vi "Test Copy Image Greyscale Mask ARGB.vi"(8 "error in (no error)":errorcluster, 11 "Test Case In":refnum<class "Image.lvclass">) -> (0 "error out":errorcluster, 3 "Test Case Out":refnum<class "Image.lvclass">)   [LabVIEW 2020, in "g_ar_toolkit.test.lvlib" / "Image.lvclass"]
uses:
  Image.lvclass
  C:/Program Files (x86)/National Instruments/LabVIEW 2020/vi.lib/Astemes/LUnit/Test Case.lvclass
  g_ar_toolkit.common/Image Size (Integer).ctl
  <vilib>/Astemes/LUnit/Test Case.lvclass/Test Case.ctl
  g_ar_toolkit.image/CreateEmptyImageGreyscale.vi
  g_ar_toolkit.image/CopyArrayToImageGreyscale.vi
  g_ar_toolkit.image/CreateEmptyImageARGB.vi
  g_ar_toolkit.image/CopyImageGreyscaleMaskARGB.vi
  4993e8ee-a06a-463a-9684-69129f64d5ce.vi
  g_ar_toolkit.image/CopyArrayToImageARGB.vi
  g_ar_toolkit.image/CreateEmptyImageGreyscale.vi/6598b9e0-8a08-46f5-91fd-ca1b87217137.vi
  g_ar_toolkit.image/CopyArrayToImageGreyscale.vi/26c70cee-9332-41f4-9755-08948a885cbe.vi
  g_ar_toolkit.image/CreateEmptyImageARGB.vi/3321fa97-f432-4e1e-8db9-a0df79aed21b.vi
  g_ar_toolkit.image/CopyImageGreyscaleMaskARGB.vi/327a14ae-2acc-4952-87c0-fab6c3cd3da3.vi
  <vilib>/Astemes/LUnit/Append Pass Result.vi
  <vilib>/Astemes/LUnit/Append Fail Result.vi
  <vilib>/Astemes/LUnit/Describe Comparison.vi
  <vilib>/Astemes/LUnit/Compare Variants.vi
  g_ar_toolkit.image/CopyArrayToImageARGB.vi/26c70cee-9332-41f4-9755-08948a885cbe.vi
  <vilib>/Astemes/LUnit/Run In UI.vi
  <vilib>/Utility/error.llb/Clear Errors.vi
  g_ar_toolkit.image/ARGBColourToU32.vi
  g_ar_toolkit.common/Module Path.vi
  <vilib>/Utility/error.llb/Error Cluster From Error Code.vi
  <vilib>/picture/pixmap.llb/Flatten Pixmap.vi
  <vilib>/Astemes/LUnit/Describe Variant.vi
  Image.lvclass/Image.ctl
  g_ar_toolkit.image/g_ar_toolkit.image.lvlib
  g_ar_toolkit.common/g_ar_toolkit.common.lvlib
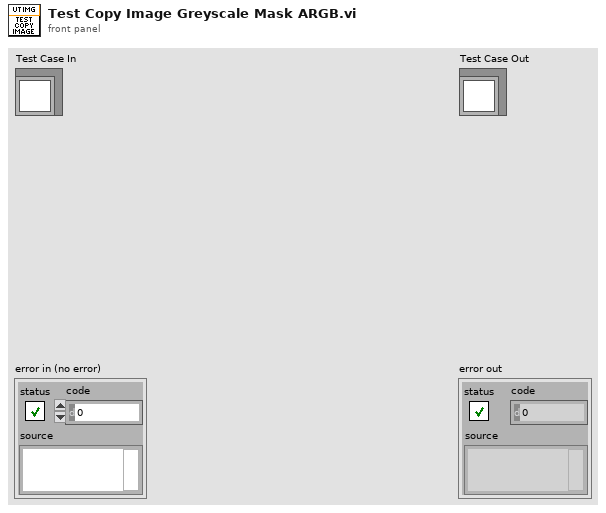
[diagram p1: front panel]
types:
  T1 = typedef "g_ar_toolkit.common.lvlib/Image Size (Integer).ctl" = cluster{"Width":u16, "Height":u16}
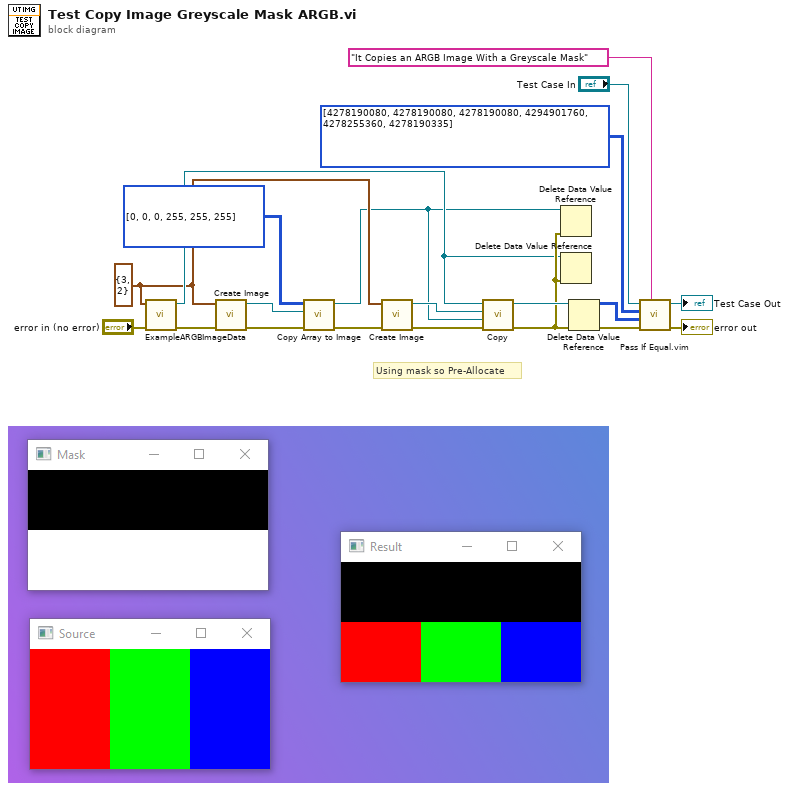
[diagram p0: block diagram]
diagram:
  w7 = T1 {"Width"=3, "Height"=2} ("Preallocated Image Size (Default - 0,0)")
  # "Using mask so Pre-Allocate"
  n1 = call "ExampleARGBImageData.vi"("error in (no error)"="error in (no error)", "Image Size"=w7) -> ("error out"=w11:errorcluster, "Data Value Reference out"=w8:refnum<data-value>)  [unwired: 6 in, 2 out]
  n2 = call-poly "Create Image.vi"("error in (no error)"=w11, "Preallocated Image Size (Default 0,0)"=w7) -> ("error out"=w15:errorcluster, "New Greyscale Image"=w4:refnum<data-value>)  [unwired: 8 in]
  n3 = call-poly "Copy Array to Image.vi"("error in (no error)"=w15, "Greyscale Destination Image"=w4, "Source"=u8[][] [[0, 0, 0], [255, 255, 255]]) -> ("error out"=w6:errorcluster, "Greyscale Destination Image (duplicate)"=w3:refnum<data-value>)  [unwired: 7 in]
  n4 = call-poly "Create Image.vi"("error in (no error)"=w6, "Preallocated Image Size (Default: 0,0)"=w7) -> ("error out"=w16:errorcluster, "New ARGB Image"=w10:refnum<data-value>)  [unwired: 8 in]
  n5 = call-poly "Copy.vi"("error in (no error)"=w16, "Greyscale Image Mask"=w3, "ARGB Image Destination"=w10, "ARGB Image Source"=w8) -> ("error out"=w9:errorcluster, "ARGB Image Destination (duplicate)"=w13:refnum<data-value>)  [unwired: 6 in]
  n6 = Delete Data Value Reference(data value reference=w3, error in=w9) -> ()  [unwired: 2 out]
  n7 = Delete Data Value Reference(data value reference=w8, error in=w9) -> ()  [unwired: 2 out]
  n8 = Delete Data Value Reference(data value reference=w13, error in=w9) -> (data value=w2:u32[][], error out=w14:errorcluster)
  n9 = call "Pass If Equal.vim"("Description"="It Copies an ARGB Image With a Greyscale Mask", "error in (no error)"=w14, "Actual"=w2, "Expected"=u32[][] [[4278190080, 4278190080, 4278190080], [4294901760, 4278255360, 4278190335]] ("data value"), "LUnit Test Case In"="Test Case In") -> ("error out"=→"error out":errorcluster, "LUnit Test Case Out"=→"Test Case Out":refnum<class "Image.lvclass">)  [unwired: 5 in]
